vi "Load Core Parallel.vi"(0 "Class Loader in":refnum<class "Class Loader.lvclass">, 5 "Caller Enqueuer":refnum<class "Message Enqueuer.lvclass">, 7 "Reference Class Path":path, 9 "Class Relative Paths Path":path, 11 "error in (no error)":errorcluster) -> (4 "Class Loader out":refnum<class "Class Loader.lvclass">, 15 "error out":errorcluster)   [LabVIEW 2023, in "Class Loader.lvlib" / "Class Loader.lvclass"]
uses:
  Class Loader.lvclass
  <vilib>/ActorFramework/Message Enqueuer/Message Enqueuer.lvclass
  Class Loader.lvclass/Class Loader.ctl
  Class Loader Messages/Class Loading Result Msg/Class Loading Result Msg.lvclass
  <vilib>/ActorFramework/Specialty Messages/Report Error Msg/Report Error Msg.lvclass
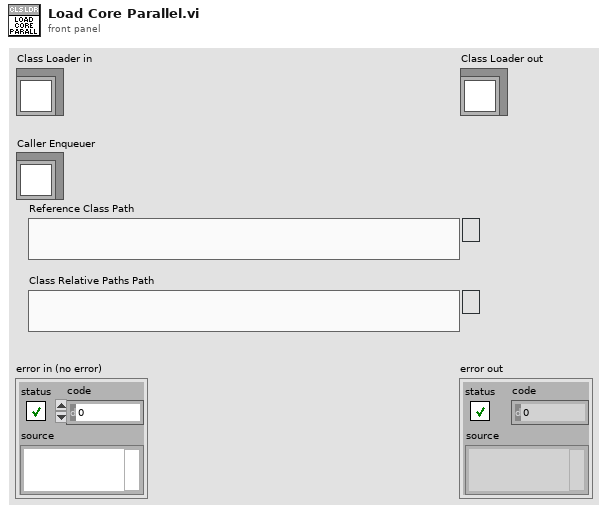
[diagram p1: front panel]
types:
  T1 = typedef "Class Loader.lvlib/Class Loader.lvclass/Classes Map.ctl" = map{string, refnum<class>}
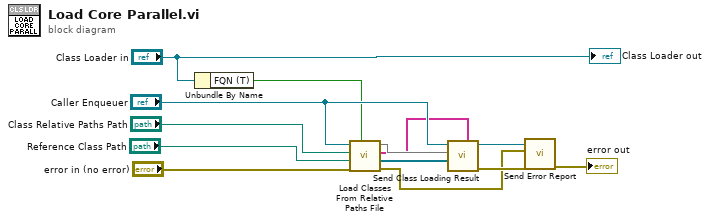
[diagram p0: block diagram]
diagram:
  n1 = Unbundle By Name("Class Loader in") -> ("FQN (T)"=w3:bool)
  n2 = call "Load Classes From Relative Paths File.vi"("FQN (T)"=w3, "error in"="error in (no error)", "Reference Class Path"="Reference Class Path", "Class Relative Paths Path"="Class Relative Paths Path", "Caller Enqueuer"="Caller Enqueuer") -> ("error out"=w5:errorcluster, "Class Array"=w8:refnum<class>[], "Class Names"=w1:string[], "Classes Map"=w2:T1)  [unwired: 3 in]
  n3 = call "Send Class Loading Result.vi"("Class Names"=w1, "Class Array"=w8, "Classes Map"=w2, "Message Enqueuer in"="Caller Enqueuer") -> ("error out"=w6:errorcluster, "Message Enqueuer out"=w7:refnum<class "Message Enqueuer.lvclass">)  [unwired: 6 in]
  n4 = call <vilib>:"Send Error Report.vi"("error in (no error)"=w6, "Error From Sender"=w5, "Message Enqueuer"=w7) -> ("error out"=→"error out":errorcluster)  [unwired: 8 in]
  "Class Loader out" <- "Class Loader in"
